vi "Run.vi"(11 "Shuwdown Event":refnum<user-event>) -> ()   [LabVIEW 2018, in "DAQmx.lvlib"]
doc: "<b>Execution System:</b> Data Acquisition"
uses:
  DAQmx.lvlib
  <vilib>/DAQmx/read.llb/DAQmx Read (Analog 2D DBL NChan NSamp).vi
  <vilib>/Analysis/baseanly.llb/Mean (DBL).vi
  <vilib>/DAQmx/read.llb/DAQmx Read (Digital 1D Bool NChan 1Samp 1Line).vi
  <vilib>/DAQmx/miscellaneous.llb/DAQmx Fill In Error Info.vi
  <vilib>/Analysis/NI_AALBase.lvlib
panel:
  out "DI Error":errorcluster
  out "AI Error":errorcluster
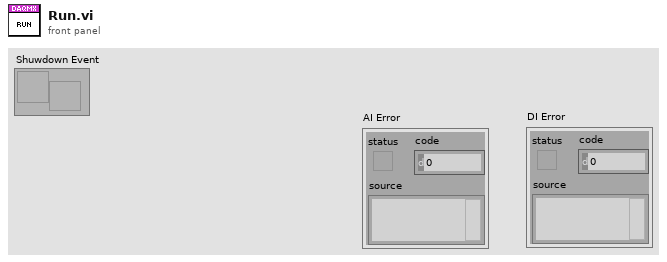
[diagram p1: front panel]
types:
  T1 = typedef "DAQmx.lvlib/DAQmx Shortcut.ctl" = cluster{"DAQmx Global Channel":refnum<k21>, "Message Queue":string, "Event":string, "Target":string, "Momentary":bool, "Data":variant}
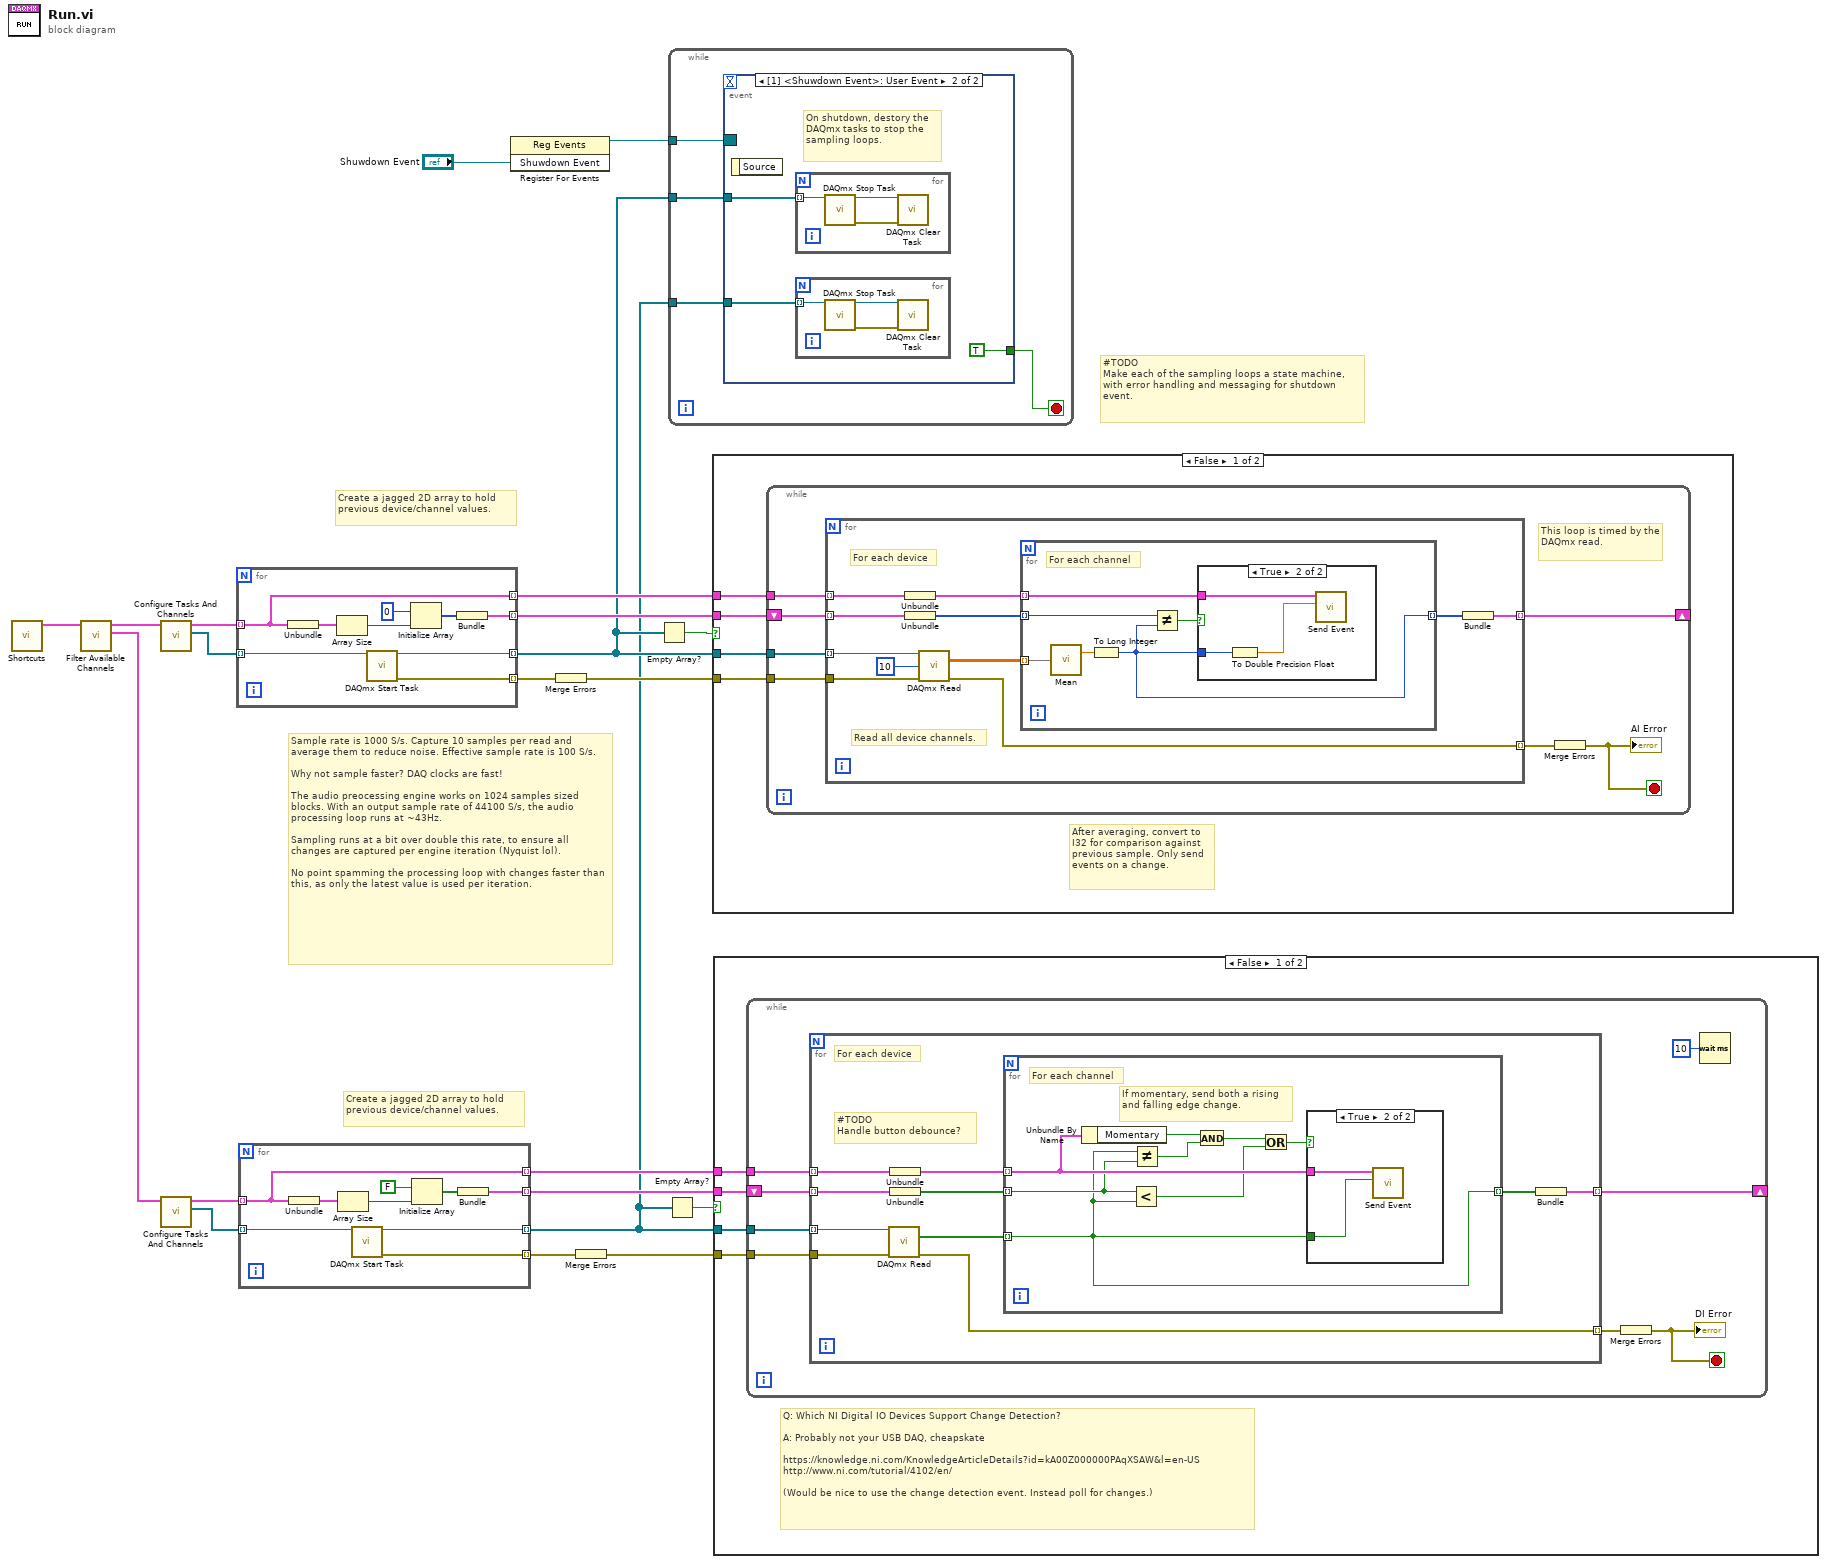
[diagram p0: block diagram]
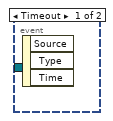
[diagram p6: hidden frame]
diagram:
  # "#TODO\nMake each of the sampling loops a state machine, with error handling and messaging for shutdown event."
  # "Create a jagged 2D array to hold previous device/channel values."
  # "Create a jagged 2D array to hold previous device/channel values."
  # "Sample rate is 1000 S/s. Capture 10 samples per read and average them to reduce noise. Effective sample rate is 100 S/s.\n\nWhy not sample faster? DAQ clocks are fast!\n\nThe audio preocessing engine works on 1024 samples sized blocks. With an output sample rate of 44100 S/s, the audio processing loop runs at ~43Hz.\n\nSampling runs at a bit over double this rate, to ensure all changes are captured per engine iteration (Nyquist lol).\n\nNo point spamming the processing loop with changes faster than this, as only the latest value is used per iteration."
  n1 = call "Shortcuts.vi"() -> ("DAQmx Shortcuts"=w6:T1[])  [unwired: 11 in]
  n2 = call "Filter Available Channels.vi"("DAQmx Shortcuts"=w6) -> ("DAQmx DI Shortcuts"=w15:T1[], "DAQmx AI Shortcuts"=w16:T1[])  [unwired: 9 in]
  n3 = call "Configure Tasks And Channels.vi"("DAQmx Shortcuts"=w16) -> ("Task Per Device"=w13:refnum<k21>[], "DAQmx Shortcuts Per Device"=w14:cluster{T1[]}[])  [unwired: 9 in]
  n4 = call "Configure Tasks And Channels.vi"("DAQmx Shortcuts"=w15) -> ("Task Per Device"=w11:refnum<k21>[], "DAQmx Shortcuts Per Device"=w12:cluster{T1[]}[])  [unwired: 9 in]
  n5 = for {
    tunnel: [w30] -> w21 mode=indexing
    tunnel: [w29] -> w20 mode=indexing
    tunnel: [w28] -> w4 mode=indexing
    tunnel: w13 -> [w27] mode=indexing
    tunnel: w14 -> [w22] mode=indexing
    tunnel: [w22] -> w17 mode=indexing
    n6 = Unbundle(w22) -> (w23:T1[])
    n7 = Array Size(array=w23) -> (size(s)=w25:i32)
    n8 = call <vilib>:"DAQmx Start Task.vi"("task/channels in"=w27) -> ("task out"=w28:refnum<k21>, "error out"=w30:errorcluster)  [unwired: 13 in]
    n9 = Initialize Array(0 ("element"), w25) -> (w24:i32[])
    n10 = Bundle(w24) -> (w29:cluster{i32[]})  [unwired: 1 in]
  }
  n11 = for {
    tunnel: [w39] -> w10 mode=indexing
    tunnel: [w38] -> w8 mode=indexing
    tunnel: [w37] -> w2 mode=indexing
    tunnel: w11 -> [w36] mode=indexing
    tunnel: w12 -> [w31] mode=indexing
    tunnel: [w31] -> w7 mode=indexing
    n12 = Unbundle(w31) -> (w32:T1[])
    n13 = Array Size(array=w32) -> (size(s)=w34:i32)
    n14 = call <vilib>:"DAQmx Start Task.vi"("task/channels in"=w36) -> ("task out"=w37:refnum<k21>, "error out"=w39:errorcluster)  [unwired: 13 in]
    n15 = Initialize Array(FALSE, w34) -> (w33:bool[])
    n16 = Bundle(w33) -> (w38:cluster{bool[]})  [unwired: 1 in]
  }
  n17 = register-events("Shuwdown Event") -> (reference out=w18:refnum<event-registration>)  [unwired: 2 in, 1 out]
  n18 = Merge Errors(w21) -> (w5:errorcluster)
  n19 = Merge Errors(w10) -> (w9:errorcluster)
  n20 = Empty Array?(array=w4) -> (empty?=w3:bool)
  n21 = Empty Array?(array=w2) -> (empty?=w1:bool)
  n22 = while {
    tunnel: w18 -> [w43]
    tunnel: w4 -> [w41]
    tunnel: w2 -> [w40]
    stop <- w42 stop-if-true
    n23 = event shown="[1] <Shuwdown Event>: User Event" {
      selector: w43 -> [_ _]
      dyn-events: _ -> [_ _]
      timeout: _ -> [_ _]
      tunnel: [_ TRUE] -> w42
      tunnel: w41 -> [_ w45]
      tunnel: w40 -> [_ w44]
      event Timeout {
        n24 = event-data() -> ()  [unwired: 1 in, 3 out]
      }
      event User Event {
        # "On shutdown, destory the DAQmx tasks to stop the sampling loops."
        n25 = event-data() -> ()  [unwired: 1 in, 1 out]
        n26 = for {
          tunnel: w45 -> [w50] mode=indexing
          n27 = call <vilib>:"DAQmx Stop Task.vi"("task/channels in"=w50) -> ("task out"=w51:refnum<k21>, "error out"=w52:errorcluster)  [unwired: 13 in]
          n28 = call <vilib>:"DAQmx Clear Task.vi"("task in"=w51, "error in"=w52) -> ()  [unwired: 13 in, 1 out]
        }
        n29 = for {
          tunnel: w44 -> [w47] mode=indexing
          n30 = call <vilib>:"DAQmx Stop Task.vi"("task/channels in"=w47) -> ("task out"=w48:refnum<k21>, "error out"=w49:errorcluster)  [unwired: 13 in]
          n31 = call <vilib>:"DAQmx Clear Task.vi"("task in"=w48, "error in"=w49) -> ()  [unwired: 13 in, 1 out]
        }
      }
    }
  }
  n32 = case shown="False" w3 {
    tunnel: w20 -> [w56 _]
    tunnel: w17 -> [w55 _]
    tunnel: w5 -> [w54 _]
    tunnel: w4 -> [w53 _]
    frame False {
      # "After averaging, convert to I32 for comparison against previous sample. Only send events on a change."
      n33 = while {
        tunnel: w53 -> [w63]
        tunnel: w54 -> [w62]
        tunnel: w55 -> [w60]
        shift-right: [w59] -> _
        shift-left: w56 -> [w61]
        stop <- w57 stop-if-true
        # "This loop is timed by the DAQmx read."
        n34 = for {
          tunnel: w63 -> [w74] mode=indexing
          tunnel: w62 -> [w73]
          tunnel: w61 -> [w66] mode=indexing
          tunnel: w60 -> [w70] mode=indexing
          tunnel: [w64] -> w59 mode=indexing
          tunnel: [w68] -> w58 mode=indexing
          # "For each device"
          # "Read all device channels."
          n35 = Unbundle(w70) -> (w65:T1[])
          n36 = Unbundle(w66) -> (w67:i32[])
          n37 = call-poly <vilib>:"DAQmx Read.vi"("task/channels in"=w74, "number of samples per channel"=10, "error in"=w73) -> ("data"=w71:dbl[][], "error out"=w68:errorcluster)  [unwired: 10 in, 1 out]
          n38 = for {
            tunnel: w71 -> [w80] mode=indexing
            tunnel: w67 -> [w79] mode=indexing
            tunnel: w65 -> [w78] mode=indexing
            tunnel: [w75] -> w69 mode=indexing
            # "For each channel"
            n39 = call-poly <vilib>:"Mean.vi"("X"=w80) -> ("mean"=w76:dbl)  [unwired: 1 out]
            n40 = To Long Integer(number=w76) -> (32bit integer=w75:i32)
            n41 = Not Equal?(x=w79, y=w75) -> (x != y?=w77:bool)
            n42 = case shown="True" w77 {
              tunnel: w78 -> [_ w82]
              tunnel: w75 -> [_ w83]
              frame False {
              }
              frame True {
                n43 = To Double Precision Float(number=w83) -> (double precision float=w81:dbl)
                n44 = call "Send Event.vi"("Data"=w81, "DAQmx Shortcut"=w82) -> ()  [unwired: 10 in]
              }
            }
          }
          n45 = Bundle(w69) -> (w64:cluster{i32[]})  [unwired: 1 in]
        }
        n46 = Merge Errors(w58) -> (w57:errorcluster)
        "AI Error" <- w57
      }
    }
    frame True {
    }
  }
  n47 = case shown="False" w1 {
    tunnel: w9 -> [w87 _]
    tunnel: w2 -> [w86 _]
    tunnel: w8 -> [w85 _]
    tunnel: w7 -> [w84 _]
    frame False {
      # "Q: Which NI Digital IO Devices Support Change Detection?\n\nA: Probably not your USB DAQ, cheapskate\n\nhttps://knowledge.ni.com/KnowledgeArticleDetails?id=kA00Z000000PAqXSAW&l=en-US\nhttp://www.ni.com/tutorial/4102/en/\n\n(Would be nice to use the change detection event. Instead poll for changes.)"
      n48 = while {
        tunnel: w87 -> [w93]
        tunnel: w86 -> [w94]
        tunnel: w84 -> [w91]
        shift-right: [w88] -> _
        shift-left: w85 -> [w92]
        stop <- w89 stop-if-true
        n49 = for {
          tunnel: w94 -> [w105] mode=indexing
          tunnel: w93 -> [w104]
          tunnel: w92 -> [w101] mode=indexing
          tunnel: w91 -> [w102] mode=indexing
          tunnel: [w98] -> w90 mode=indexing
          tunnel: [w96] -> w88 mode=indexing
          # "#TODO\nHandle button debounce?"
          # "For each device"
          n50 = call-poly <vilib>:"DAQmx Read.vi"("task/channels in"=w105, "error in"=w104) -> ("data"=w103:bool[], "error out"=w98:errorcluster)  [unwired: 11 in, 1 out]
          n51 = Unbundle(w102) -> (w100:T1[])
          n52 = Unbundle(w101) -> (w99:bool[])
          n53 = for {
            tunnel: w103 -> [w108] mode=indexing
            tunnel: w100 -> [w112] mode=indexing
            tunnel: w99 -> [w109] mode=indexing
            tunnel: [w108] -> w97 mode=indexing
            # "If momentary, send both a rising and falling edge change."
            # "For each channel"
            n54 = Unbundle By Name(w112) -> ("Momentary"=w111:bool)
            n55 = Less?(x=w109, y=w108) -> (x < y?=w107:bool)
            n56 = Not Equal?(x=w108, y=w109) -> (x != y?=w113:bool)
            n57 = And(x=w111, y=w113) -> (x .and. y?=w110:bool)
            n58 = Or(x=w110, y=w107) -> (x .or. y?=w106:bool)
            n59 = case shown="True" w106 {
              tunnel: w112 -> [_ w115]
              tunnel: w108 -> [_ w114]
              frame False {
              }
              frame True {
                n60 = call "Send Event.vi"("Data"=w114, "DAQmx Shortcut"=w115) -> ()  [unwired: 10 in]
              }
            }
          }
          n61 = Bundle(w97) -> (w96:cluster{bool[]})  [unwired: 1 in]
        }
        n62 = Merge Errors(w90) -> (w89:errorcluster)
        "DI Error" <- w89
        n63 = Wait (ms)(milliseconds to wait=u32 10) -> ()  [unwired: 1 out]
      }
    }
    frame True {
    }
  }
